vi "LB_GetFirmwareversion.vi"(8 "error in (no error)":errorcluster caption="错误输入（无错误）", 11 "LB_COM_IN":refnum<visa-resource-name>="COM4") -> (0 "error out":errorcluster caption="错误输出", 2 "OK":bool, 3 "LB_COM_OUT":refnum<visa-resource-name>)   [LabVIEW 2015, in "LBAnalyser.lvlib"]
uses:
  LBAnalyser.lvlib
  UartCOM/UARTCOM.lvlib
panel:
  out "读取字符串":string
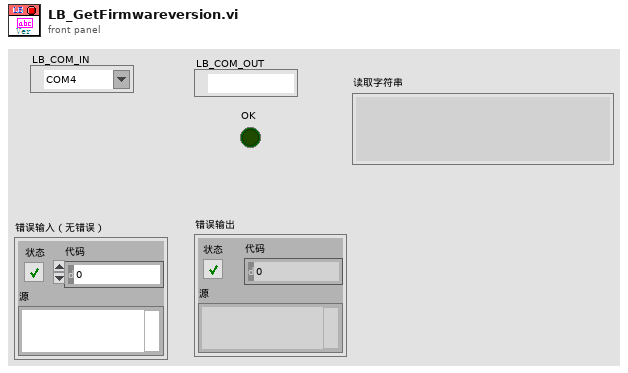
[diagram p1: front panel]
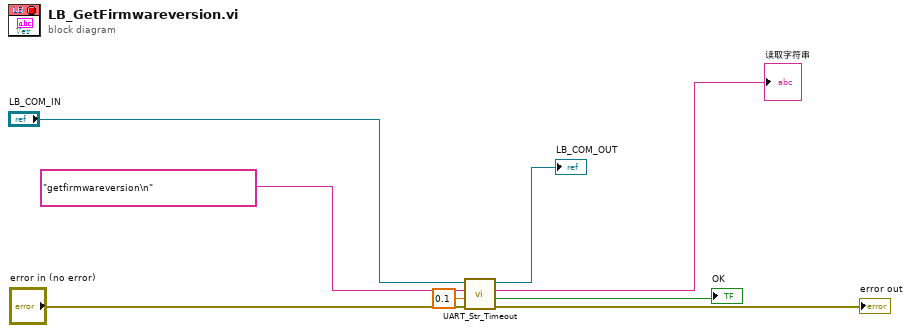
[diagram p0: block diagram]
diagram:
  n1 = call "UART_Str_Timeout.vi"("error in (no error)"="error in (no error)", "超时s"=0.1, "写入字符串"="getfirmwareversion\n", "BASE_COM"="LB_COM_IN") -> ("error out"=→"error out":errorcluster, "OK"=→"OK":bool, "读取字符串"=→"读取字符串":string, "BASE_COM_OUT"=→"LB_COM_OUT":refnum<visa-resource-name>)  [unwired: 3 in, 1 out]
